vi "FrequencyDomainCorrelationArrays.vi"(10 "Template":u8[][](array[numeric]), 11 "Image":u8[][](array[numeric])) -> (3 "FDCorrelation":dbl[][](array[numeric]))   [LabVIEW 2014]
uses:
  <vilib>/Analysis/2dsp.llb/2D Real FFT.vi
  <vilib>/Analysis/2dsp.llb/2D Inverse Real FFT.vi
  <vilib>/Analysis/NI_AALPro.lvlib
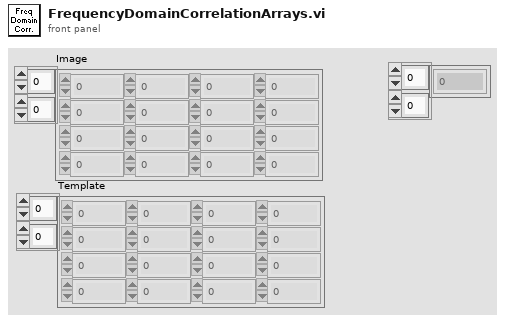
[diagram p1: front panel]
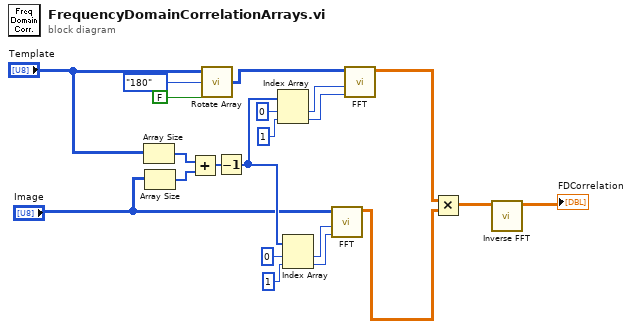
[diagram p0: block diagram]
diagram:
  n1 = Array Size(array="Template") -> (size(s)=w21:i32[])
  n2 = Array Size(array="Image") -> (size(s)=w20:i32[])
  n3 = Add(x=w21, y=w20) -> (x+y=w19:i32[])
  n4 = call "Rotate Array.vi"("Rotation Orientation"=FALSE, "Rotation"=enum8{"90", "180", "270"}."180", "Array"="Template") -> ("Rotated 2D Array"=w1:u8[][])
  n5 = Decrement(x=w19) -> (x-1=w12:i32[])
  n6 = Index Array(array=w12, index #1=0 ("index"), index #2=1 ("index")) -> (element #1=w16:i32, element #2=w15:i32)
  n7 = Index Array(array=w12, index #1=0 ("index"), index #2=1 ("index")) -> (element #1=w11:i32, element #2=w10:i32)
  n8 = call-poly <vilib>:"FFT.vi"("n"=w10, "m"=w11, "X"="Image") -> ("FFT {X}"=w8:cdb[][])  [unwired: 7 in, 1 out]
  n9 = call-poly <vilib>:"FFT.vi"("n"=w15, "m"=w16, "X"=w1) -> ("FFT {X}"=w9:cdb[][])  [unwired: 7 in, 1 out]
  n10 = Multiply(x=w9, y=w8) -> (x*y=w7:cdb[][])
  n11 = call-poly <vilib>:"Inverse FFT.vi"("FFT {X}"=w7) -> ("X"=→"FDCorrelation":dbl[][])  [unwired: 9 in, 1 out]
